vi "Write Warning_.vi"(8 "error in (no error)":errorcluster, 10 "Warning?":bool, 11 "AssertError in":refnum<class "AssertError.lvclass">) -> (0 "error out":errorcluster, 3 "AssertError out":refnum<class "AssertError.lvclass">)   [LabVIEW 2021, in "Bananas.lvlib" / "AssertError.lvclass"]
uses:
  AssertError.lvclass
  AssertError.lvclass/AssertError.ctl
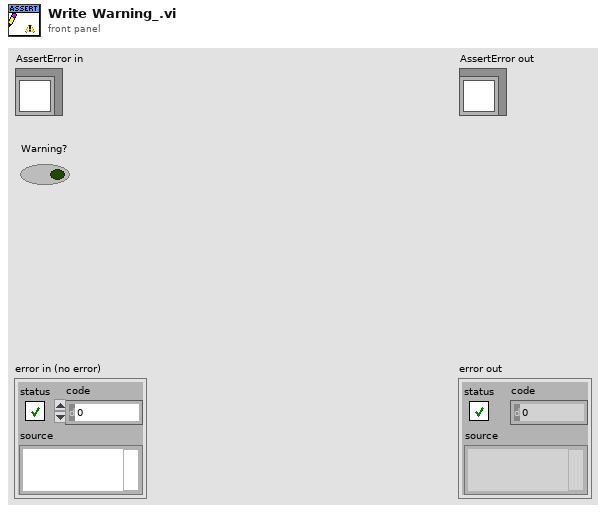
[diagram p1: front panel]
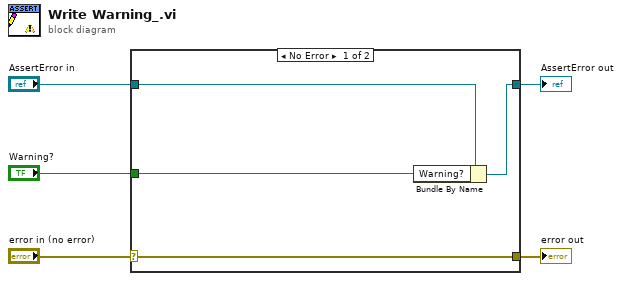
[diagram p0: block diagram]
diagram:
  n1 = case shown="No Error" "error in (no error)" {
    selector: "error in (no error)" -> [w9 w10]
    tunnel: [w9 w10] -> w4
    tunnel: [w7 w11] -> w2
    tunnel: "AssertError in" -> [w8 w11]
    tunnel: "Warning?" -> [w6 _]
    frame No Error {
      n2 = Bundle By Name(cluster=w8, "Warning?"=w6) -> (w7:refnum<class "AssertError.lvclass">)
    }
    frame Error {
    }
  }
  "error out" <- w4
  "AssertError out" <- w2
